vi "Get_Packet_TDMS_Information.vi"() -> (1 "TDMS Info 5Hz":T1={"All Data Types"=[], "All Units"=[], "All Names"=[], "Group Name"="5Hz"}, 3 "TDMS Info 50Hz":T1={"All Data Types"=[], "All Units"=[], "All Names"=[], "Group Name"="50Hz"})   [LabVIEW 2019, in "SpatialDual_Parsers.lvlib"]
uses:
  SpatialDual_Parsers.lvlib
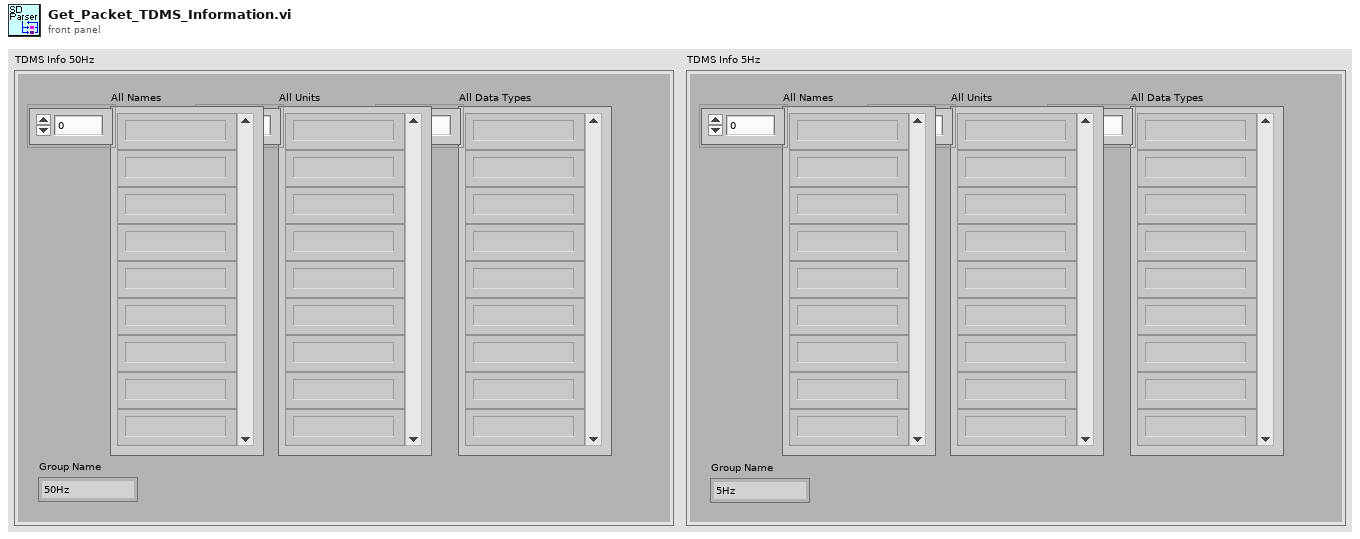
[diagram p1: front panel]
types:
  T1 = cluster{"All Data Types":string[], "All Units":string[], "All Names":string[], "Group Name":string}
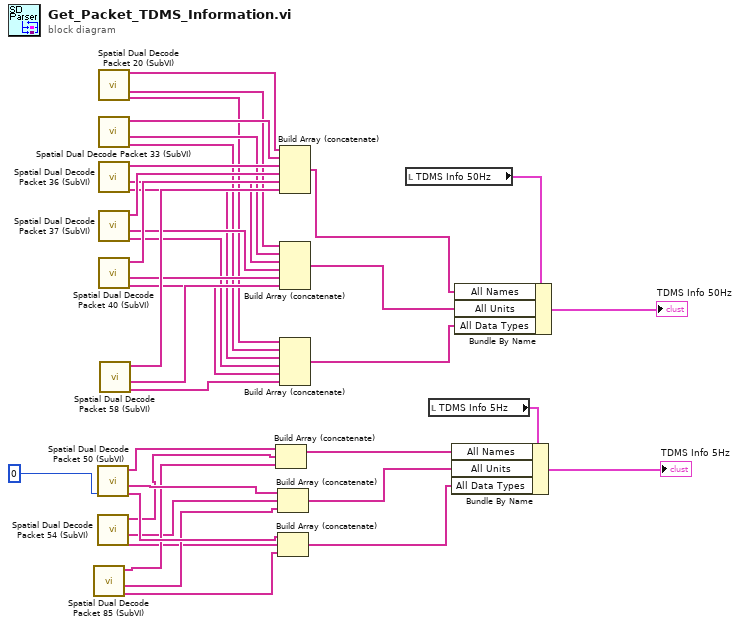
[diagram p0: block diagram]
diagram:
  n1 = call "Spatial Dual Decode Packet 85 (SubVI).vi"() -> ("Channel Data Type"=w2:string[], "Channel Units"=w4:string[], "Channel Names"=w6:string[])  [unwired: 6 in, 2 out]
  n2 = call "Spatial Dual Decode Packet 50 (SubVI).vi"("Unix Timestamp"=u64 0) -> ("Channel Data Type"=w13:string[], "Channel Units"=w14:string[], "Channel Names"=w15:string[])  [unwired: 5 in, 2 out]
  n3 = call "Spatial Dual Decode Packet 54 (SubVI).vi"() -> ("Channel Data Type"=w3:string[], "Channel Units"=w5:string[], "Channel Names"=w7:string[])  [unwired: 6 in, 2 out]
  n4 = call "Spatial Dual Decode Packet 20 (SubVI).vi"() -> ("Channel Names"=w38:string[], "Channel Units"=w27:string[], "Data Types"=w21:string[])  [unwired: 10 in, 3 out]
  n5 = call "Spatial Dual Decode Packet 33 (SubVI).vi"() -> ("Channel Data Type"=w22:string[], "Channel Units"=w28:string[], "Channel Names"=w37:string[])  [unwired: 6 in, 2 out]
  n6 = call "Spatial Dual Decode Packet 36 (SubVI).vi"() -> ("Channel Data Type"=w23:string[], "Channel Units"=w29:string[], "Channel Names"=w36:string[])  [unwired: 6 in, 2 out]
  n7 = call "Spatial Dual Decode Packet 37 (SubVI).vi"() -> ("Channel Data Type"=w24:string[], "Channel Units"=w30:string[], "Channel Names"=w35:string[])  [unwired: 6 in, 2 out]
  n8 = call "Spatial Dual Decode Packet 40 (SubVI).vi"() -> ("Channel Data Type"=w25:string[], "Channel Units"=w31:string[], "Channel Names"=w34:string[])  [unwired: 6 in, 2 out]
  n9 = call "Spatial Dual Decode Packet 58 (SubVI).vi"() -> ("Channel Data Type"=w26:string[], "Channel Units"=w32:string[], "Channel Names"=w33:string[])  [unwired: 6 in, 2 out]
  n10 = Build Array (concatenate)(w15, w7, w6) -> (w11:string[])
  n11 = Build Array (concatenate)(w14, w5, w4) -> (w10:string[])
  n12 = Build Array (concatenate)(w13, w3, w2) -> (w9:string[])
  n13 = Build Array (concatenate)(w38, w37, w36, w35, w34, w33) -> (w20:string[])
  n14 = Build Array (concatenate)(w27, w28, w29, w30, w31, w32) -> (w19:string[])
  n15 = Build Array (concatenate)(w21, w22, w23, w24, w25, w26) -> (w18:string[])
  n16 = local read "TDMS Info 50Hz"() -> (w16:T1)
  n17 = local read "TDMS Info 5Hz"() -> (w12:T1)
  n18 = Bundle By Name(cluster=w12, "All Names"=w11, "All Units"=w10, "All Data Types"=w9) -> (→"TDMS Info 5Hz":T1)
  n19 = Bundle By Name(cluster=w16, "All Names"=w20, "All Units"=w19, "All Data Types"=w18) -> (→"TDMS Info 50Hz":T1)
